vi "ReleaseNotifiers.vi"(8 "error in (no error)":errorcluster, 11 "DAQmx":refnum<class "DAQmx.lvclass">) -> (0 "error out":errorcluster, 3 "DAQmx out":refnum<class "DAQmx.lvclass">)   [LabVIEW 2019, in "DAQmx.lvclass"]
uses:
  DAQmx.lvclass
  DAQmx.lvclass/DAQmx.ctl
panel:
  # "For instructions on how to use the JKI State Machine Objects, examples and video tutorials, visit:\nhttp://jki.net/state-machine-objects/\n\nJKI State Machine Objects™\nhttp://jki.net/state-machine-objects/\nCopyright (C) 2005-2015, JKI <info@jki.net>\nALL RIGHTS RESERVED"
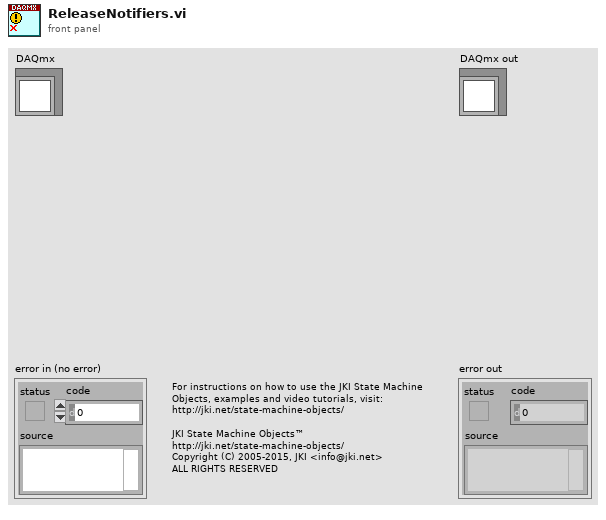
[diagram p1: front panel]
types:
  T1 = typedef "DAQmx.lvclass/PrivateQueues--Cluster.ctl" = cluster{"Action":refnum<queue>, "Timing":refnum<queue>, "AOconfig":refnum<queue>, "AIconfig":refnum<queue>}
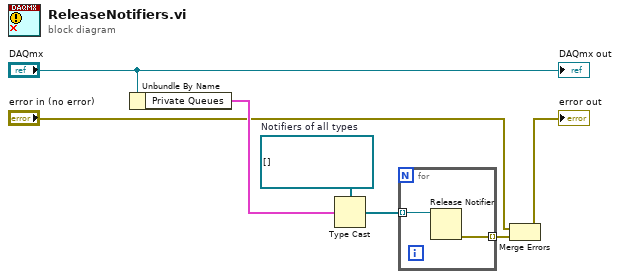
[diagram p0: block diagram]
diagram:
  w6 = refnum<notifier>[] []  # Notifiers of all types
  n1 = Unbundle By Name("DAQmx") -> ("Private Queues"=w3:T1)
  n2 = Type Cast(type=w6, x=w3) -> (*(type *) &x=w7:refnum<notifier>[])
  n3 = for {
    tunnel: w7 -> [w8] mode=indexing
    tunnel: [w9] -> w5 mode=indexing
    n4 = Release Notifier(notifier=w8) -> (error out=w9:errorcluster)  [unwired: 2 in, 2 out]
  }
  n5 = Merge Errors("error in (no error)", w5) -> (→"error out":errorcluster)
  "DAQmx out" <- "DAQmx"
